vi "Save and Recall Instrument State.vi"(8 "error in (no error)":errorcluster, 10 "State Operation (0: Save)":i32(ring) items=["Save", "Recall"], 11 "VISA resource name":refnum<visa-resource-name>) -> (0 "error out":errorcluster, 3 "VISA resource name out":refnum<visa-resource-name>)   [LabVIEW 2020, in "Agilent 34405.lvlib"]
doc: "Stores the current instrument state in the specified storage location or recalls the instrument state stored in the specified storage location."
uses:
  <instrlib>/Agilent 34405/Agilent 34405.lvlib
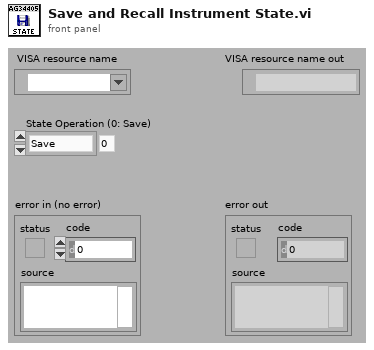
[diagram p1: front panel]
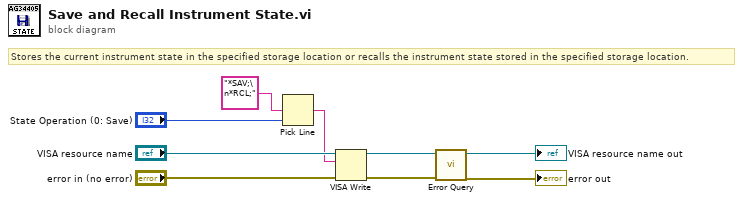
[diagram p0: block diagram]
diagram:
  # "Stores the current instrument state in the specified storage location or recalls the instrument state stored in the specified storage location."
  n1 = Pick Line(multi-line string="*SAV;\n*RCL;", line index="State Operation (0: Save)") -> (output string=w1:string)  [unwired: 1 out]
  n2 = VISA Write(VISA resource name="VISA resource name", write buffer=w1, error in (no error)="error in (no error)") -> (VISA resource name out=w7:refnum<visa-resource-name>, error out=w6:errorcluster)  [unwired: 1 out]
  n3 = call <instrlib>:"Error Query.vi"("error in (no error)"=w6, "VISA resource name"=w7) -> ("error out"=→"error out":errorcluster, "VISA resource name out"=→"VISA resource name out":refnum<visa-resource-name>)  [unwired: 8 out]
